vi "crd_acquireWaveform.vi"(6 "Max Adc value":i16, 8 "error in (no error)":errorcluster, 9 "Device Info":T2, 10 "handle":i16, 11 "Queue in":refnum<queue>) -> (0 "error out":errorcluster, 2 "handle out":i16, 3 "Queue out":refnum<queue>)   [LabVIEW 2011]
panel:
  in  "Acquisition Settings":T1={"preTriggerSamples"=0, "postTriggerSamples"=11000, "timebase"=4, "Down-Sample Mode"=0, "Down Sample Ratio"=1, "Oversample"=1} {"Down-Sample Mode" items=["None"=0, "Aggregate"=1, "Decimate"=2, "Average"=4]}
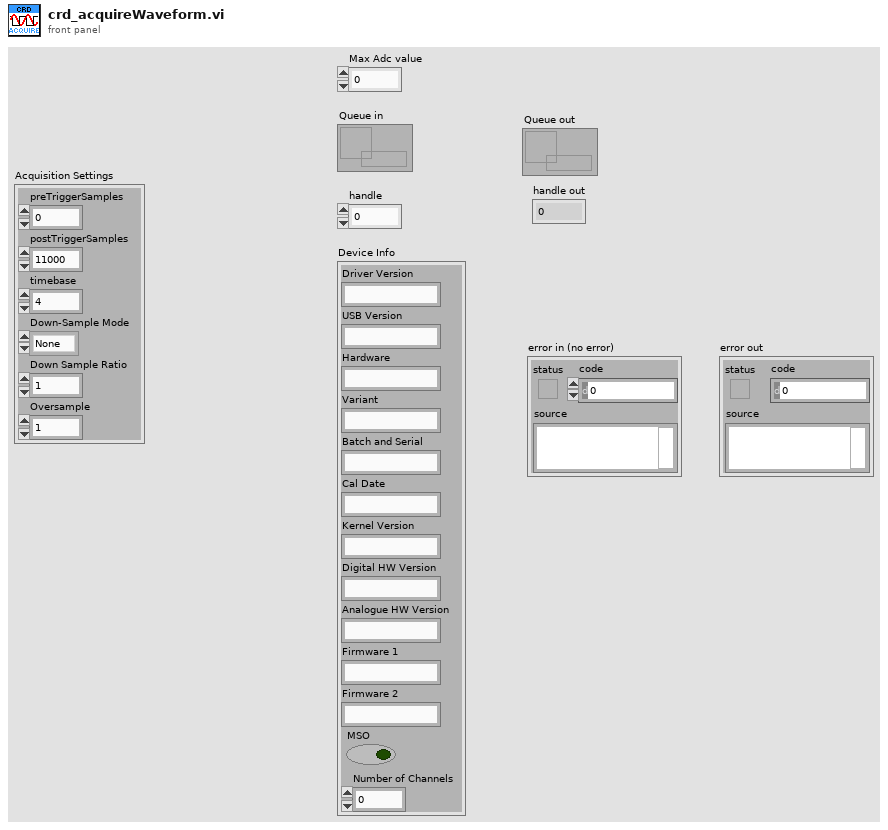
[diagram p1: front panel]
types:
  T1 = cluster{"preTriggerSamples":u32, "postTriggerSamples":u32, "timebase":u32, "Down-Sample Mode":i32, "Down Sample Ratio":u32, "Oversample":i16}
  T2 = cluster{"Driver Version":string, "USB Version":string, "Hardware":string, "Variant":string, "Batch and Serial":string, "Cal Date":string, "Kernel Version":string, "Digital HW Version":string, "Analogue HW Version":string, "Firmware 1":string, "Firmware 2":string, "MSO":bool, "Number of Channels":i16}
  T3 = cluster{"Enabled":bool, "Coupling":i16, "Range":u16, "Analogue Offset":sgl}
  T4 = cluster{"Trigger Enabled":bool, "Trigger Source":enum16{"Channel A", "Channel B", "Channel C", "Channel D", "Ext."}, "Trigger Threshold (Volts)":dbl, "Trigger Direction":u16, "Trigger Delay (samples)":u32, "Auto Trigger Time (ms)":i16}
  T5 = cluster{"Sample Frequency":sgl, "Sample Internal":sgl, "Max Samples Available":i32, "Number of Samples":u32, "Total Capture Time (sec) ":sgl, "Max Total Capture Time Available (sec)":sgl}
  T6 = cluster{"Channel D Buffer":i16[], "Channel C Buffer":i16[], "Channel B Buffer":i16[], "Channel A Buffer":i16[], "Port 0  Buffer ":i16[], "Port 1 Buffer ":i16[]}
  T7 = cluster{i32, "Sample Internal":sgl, "Data (Volts)":dbl[]}
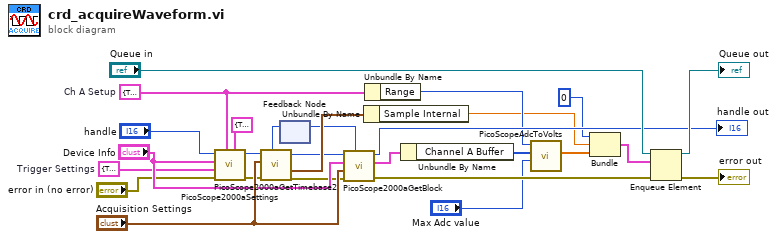
[diagram p0: block diagram]
diagram:
  w4 = T3 {"Enabled"=TRUE, "Coupling"=1, "Range"=3, "Analogue Offset"=0.0}  # Ch A Setup
  w5 = T4 {"Trigger Enabled"=TRUE, "Trigger Source"=enum."Channel B", "Trigger Threshold (Volts)"=0.35, "Trigger Direction"=3, "Trigger Delay (samples)"=0, "Auto Trigger Time (ms)"=1000}  # Trigger Settings
  n1 = call "PicoScope2000aSettings.vi"("Channel B Settings"=T3 {"Enabled"=TRUE, "Coupling"=0, "Range"=7, "Analogue Offset"=0.0}, "Channel A Settings"=w4, "error in"="error in (no error)", "Trigger Settings"=w5, "Device Info"="Device Info", "handle in"="handle") -> ("error out"=w11:errorcluster, "handle out"=w10:i16)  [unwired: 4 in]
  n2 = feedback #1() -> (w13:u32)  [unwired: 1 in]
  n3 = call "PicoScope2000aGetTimebase2.vi"("Number of Samples"=w13, "error in (no error)"=w11, "Acquisition Settings"="Acquisition Settings", "handle in"=w10) -> ("error out"=w14:errorcluster, "Properties Panel"=w17:T5, "handle out"=w15:i16)  [unwired: 5 in]
  n4 = call "PicoScope2000aGetBlock.vi"("error in"=w14, "Acquisition Settings"="Acquisition Settings", "Device Info"="Device Info", "handle in"=w15) -> ("error out"=w26:errorcluster, "Buffers (Max or non-aggregated)"=w18:T6, "handle out"=→"handle out":i16, "noOfSamples"=w12:u32)  [unwired: 2 in, 2 out]
  n5 = feedback-in #1(w12) -> ()
  n6 = Unbundle By Name(w17) -> ("Sample Internal"=w3:sgl)
  n7 = Unbundle By Name(w4) -> ("Range"=w8:u16)
  n8 = Unbundle By Name(w18) -> ("Channel A Buffer"=w19:i16[])
  n9 = call "PicoScopeAdcToVolts.vi"("Max_adc"="Max Adc value", "Data"=w19, "Range Index"=w8) -> ("Data (Volts)"=w2:dbl[])  [unwired: 8 in]
  n10 = Bundle(0, "Sample Internal"=w3, "Data (Volts)"=w2) -> (w24:T7)  [unwired: 1 in]
  n11 = Enqueue Element(queue="Queue in", element=w24, error in (no error)=w26) -> (queue out=→"Queue out":refnum<queue>, error out=→"error out":errorcluster)  [unwired: 1 in, 1 out]
